vi "CreateSingleQueue.vi"(8 "Error In":errorcluster, 11 "Number of Queues":i32) -> (0 "Error Out":errorcluster, 3 "Q_MEMs":refnum<queue>[](array[refnum]))   [LabVIEW 2014]
uses:
  02_Controls/Message_Data_Ctl.ctl
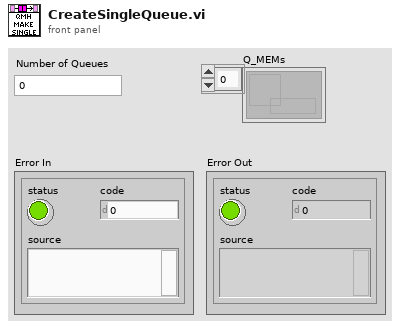
[diagram p1: front panel]
types:
  T1 = typedef "Message_Data_Ctl.ctl" = cluster{"Message":string, "Data":variant}
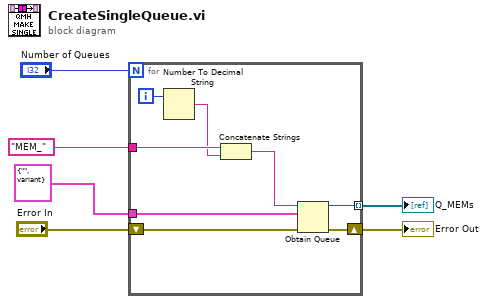
[diagram p0: block diagram]
diagram:
  n1 = for {
    N: "Number of Queues" -> [_]
    tunnel: T1 {"Message"="", "Data"=variant} ("Message_Data") -> [w12]
    tunnel: [w11] -> w1 mode=indexing
    shift-right: [w13] -> w5
    shift-left: "Error In" -> [w14]
    tunnel: "MEM_" -> [w9]
    i -> [w10]
    n2 = Number To Decimal String(number=w10) -> (decimal integer string=w8:string)  [unwired: 1 in]
    n3 = Concatenate Strings(w9, w8) -> (w7:string)
    n4 = Obtain Queue(name (unnamed)=w7, element data type=w12, error in (no error)=w14) -> (queue out=w11:refnum<queue>, error out=w13:errorcluster)  [unwired: 2 in, 1 out]
  }
  "Error Out" <- w5
  "Q_MEMs" <- w1
